vi "主程序.vi"() -> ()   [LabVIEW 2010]
panel:
  out "the average should be equal to":dbl
  out "average of random numbers":dbl
  out "iteration counter":dbl
  in  "?":dbl(slide) scale=0.0..1000.0
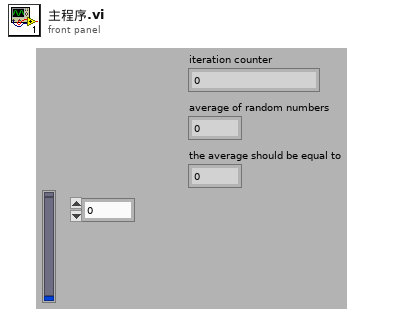
[diagram p1: front panel]
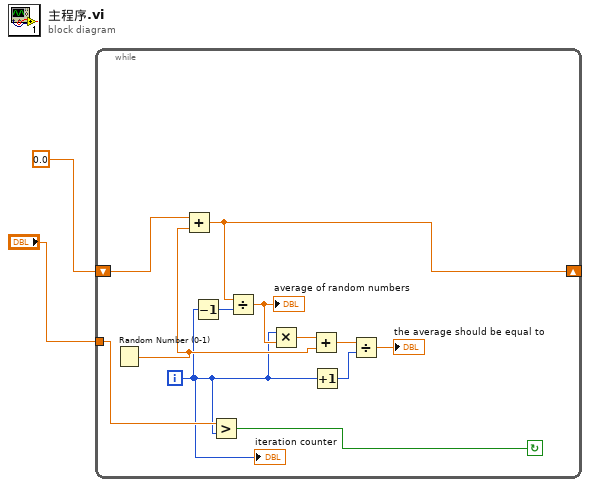
[diagram p0: block diagram]
diagram:
  n1 = while {
    shift-right: [w13] -> _
    shift-left: 0.0 -> [w14]
    tunnel: "?" -> [w5]
    i -> [w3]
    stop <- w4 continue-if-true
    n2 = Random Number (0-1)() -> (number: 0 to 1=w6:dbl)
    n3 = Add(x=w14, y=w6) -> (x+y=w13:dbl)
    n4 = Decrement(x=w3) -> (x-1=w12:i32)
    n5 = Greater?(x=w5, y=w3) -> (0:w4:bool)
    n6 = Divide(x=w13, y=w12) -> (x/y=w11:dbl)
    "average of random numbers" <- w11
    n7 = Multiply(x=w3, y=w11) -> (x*y=w10:dbl)
    n8 = Add(x=w10, y=w6) -> (x+y=w9:dbl)
    n9 = Increment(x=w3) -> (x+1=w8:i32)
    n10 = Divide(x=w9, y=w8) -> (x/y=→"the average should be equal to":dbl)
    "iteration counter" <- w3
  }
